vi "Compute DistanceToTarget (Modified).vi"(8 "Y Image Resolution":i32=120, 9 "X Image Resolution":i32=160, 10 "Vertical Strip":T1, 11 "Camera Type":enum16{"206", "1011", "1013"}(ring)=enum."1011") -> (0 "Distance to Wall (ft)":dbl, 2 "Target Center (-1 to 1)":cluster{"X":dbl, "Y":dbl}, 3 "Distance to Goal Wall (ft)":dbl)   [LabVIEW 2013]
doc: "Using the camera lens information and the real world size of the target, use trig and ratios to determine the distance to the target. Also returns the location relative to the image center in a (-1 , 1) coordinate system that may be useful for steering the robot."
panel:
  in  "Slope correction (goal wall)":dbl=0.365
  in  "Offset (goal wall)":dbl=0.889
  in  "Slope correction":dbl=0.87
  in  "Offset":dbl=0.835
  in  "Camera view angles":dbl[](array[numeric])=[41.7, 37.4, 49.0]
  # "37.4 default for M1011"
  # "Axis 206\nAxis M1011\nAxis M1013"
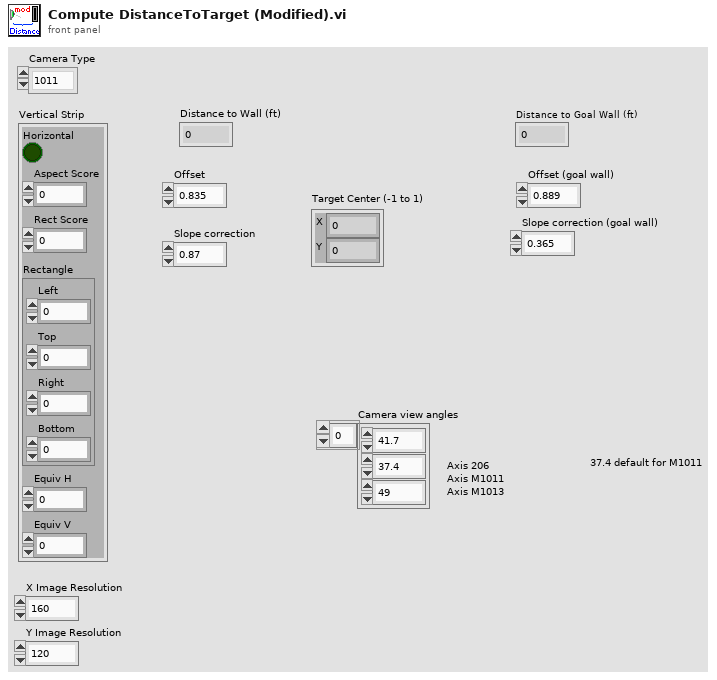
[diagram p1: front panel]
types:
  T1 = cluster{"Horizontal":bool, "Aspect Score":dbl, "Rect Score":dbl, "Rectangle":cluster{"Left":dbl, "Top":dbl, "Right":dbl, "Bottom":dbl}, "Equiv H":dbl, "Equiv V":dbl}
  T2 = cluster{"X Image Resolution":i32, "Y Image Resolution":i32}
  T3 = cluster{"X Image Resolution":dbl, "Y Image Resolution":dbl}
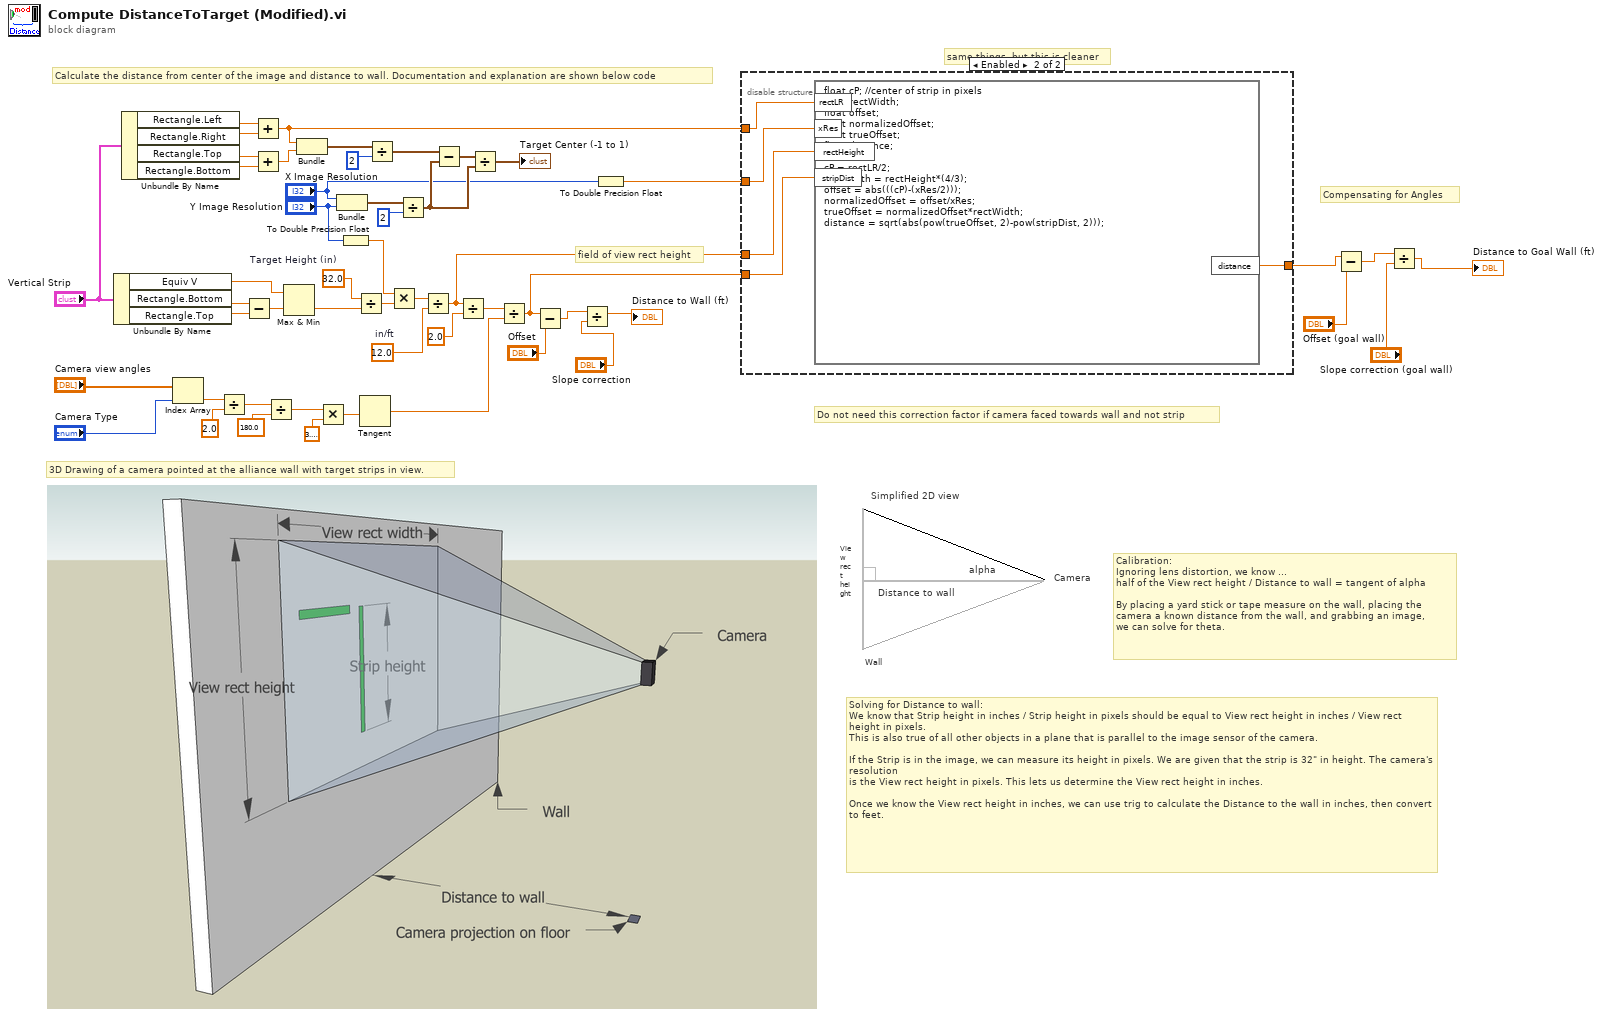
[diagram p0: block diagram]
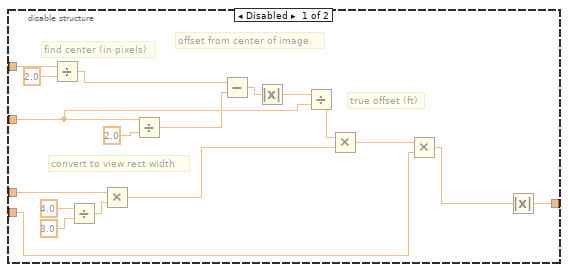
[diagram p2: hidden frame]
diagram:
  w21 = 12.0  # in/ft
  w25 = 32.0  # Target Height (in)
  # "Do not need this correction factor if camera faced towards wall and not strip"
  # "Compensating for Angles"
  # "same things, but this is cleaner"
  # "field of view rect height"
  # "Wall"
  # "Camera"
  # "Simplified 2D view"
  # "Solving for Distance to wall:\nWe know that Strip height in inches / Strip height in pixels should be equal to View rect height in inches / View rect height in pixels.\nThis is also true of all other objects in a plane that is parallel to the image sensor of the camera.\n\nIf the Strip is in the image, we can measure its height in pixels. We are given that the strip is 32\" in height. The camera's resolution\nis the View rect height in pixels. This lets us determine the View rect height in inches.\n\nOnce we know the View rect height in inches, we can use trig to calculate the Distance to the wall in inches, then convert to feet."
  # "3D Drawing of a camera pointed at the alliance wall with target strips in view."
  # "Distance to wall"
  # "View rect height"
  # "alpha"
  # "Calibration:\nIgnoring lens distortion, we know ...\nhalf of the View rect height / Distance to wall = tangent of alpha\n\nBy placing a yard stick or tape measure on the wall, placing the\ncamera a known distance from the wall, and grabbing an image,\nwe can solve for theta."
  # "Calculate the distance from center of the image and distance to wall. Documentation and explanation are shown below code"
  n1 = Unbundle By Name("Vertical Strip") -> ("Equiv V"=w27:dbl, "Rectangle.Bottom"=w42:dbl, "Rectangle.Top"=w41:dbl)
  n2 = Unbundle By Name("Vertical Strip") -> ("Rectangle.Left"=w36:dbl, "Rectangle.Right"=w37:dbl, "Rectangle.Top"=w39:dbl, "Rectangle.Bottom"=w38:dbl)
  n3 = Index Array(array="Camera view angles", index="Camera Type") -> (element=w48:dbl)
  n4 = Divide(x=w48, y=2.0) -> (x/y=w45:dbl)
  n5 = Subtract(x=w42, y=w41) -> (x-y=w26:dbl)
  n6 = Add(x=w36, y=w37) -> (x+y=w14:dbl)
  n7 = Add(x=w39, y=w38) -> (x+y=w34:dbl)
  n8 = Divide(x=w45, y=180.0) -> (x/y=w44:dbl)
  n9 = Max & Min(x=w27, y=w26) -> (min(x,y)=w10:dbl)  [unwired: 1 out]
  n10 = Bundle(w14, w34) -> (w31:cluster{dbl, dbl})  [unwired: 1 in]
  n11 = Multiply(x=w44, y=3.141592653589793) -> (x*y=w46:dbl)
  n12 = Bundle("X Image Resolution"="X Image Resolution", "Y Image Resolution"="Y Image Resolution") -> (w33:T2)  [unwired: 1 in]
  n13 = To Double Precision Float(number="Y Image Resolution") -> (double precision float=w11:dbl)
  n14 = Divide(x=w25, y=w10) -> (x/y=w24:dbl)
  n15 = Tangent(1:w46) -> (0:w18:dbl)
  n16 = Divide(x=w31, y=2) -> (x/y=w17:cluster{dbl, dbl})
  n17 = Multiply(x=w11, y=w24) -> (x*y=w22:dbl)
  n18 = Divide(x=w33, y=2) -> (x/y=w29:T3)
  n19 = Divide(x=w22, y=w21) -> (x/y=w15:dbl)
  n20 = Subtract(x=w17, y=w29) -> (x-y=w30:cluster{dbl, dbl})
  n21 = Divide(x=w15, y=2.0) -> (x/y=w19:dbl)
  n22 = Divide(x=w30, y=w29) -> (x/y=→"Target Center (-1 to 1)":cluster{dbl, dbl})
  n23 = Divide(x=w19, y=w18) -> (x/y=w12:dbl)
  n24 = Subtract(x=w12, y="Offset") -> (x-y=w7:dbl)
  n25 = Divide(x=w7, y="Slope correction") -> (x/y=→"Distance to Wall (ft)":dbl)
  n26 = To Double Precision Float(number="X Image Resolution") -> (double precision float=w13:dbl)
  n27 = disable-structure shown="Enabled" {
    disable-tunnel: [w52 w71] -> w5
    disable-tunnel: w15 -> [w57 w73]
    disable-tunnel: w14 -> [w56 w74]
    disable-tunnel: w13 -> [w55 w72]
    disable-tunnel: w12 -> [w53 w70]
    frame Disabled {
      # "true offset (ft)"
      # "offset from center of image"
      # "find center (in pixels)"
      # "convert to view rect width"
      n28 = Divide(x=w56, y=2.0) -> (x/y=w58:dbl)
      n29 = Divide(x=4.0, y=3.0) -> (x/y=w69:dbl)
      n30 = Multiply(x=w57, y=w69) -> (x*y=w65:dbl)
      n31 = Divide(x=w55, y=2.0) -> (x/y=w63:dbl)
      n32 = Subtract(x=w58, y=w63) -> (x-y=w62:dbl)
      n33 = Absolute Value(x=w62) -> (abs(x)=w61:dbl)
      n34 = Divide(x=w61, y=w55) -> (x/y=w59:dbl)
      n35 = Multiply(x=w59, y=w65) -> (x*y=w60:dbl)
      n36 = Multiply(x=w60, y=w53) -> (x*y=w54:dbl)
      n37 = Absolute Value(x=w54) -> (abs(x)=w52:dbl)
    }
    frame Enabled {
      n38 = formula code="float cP; //center of strip in pixels\nfloat rectWidth;\nfloat offset;\nfloat normalizedOffset;\nfloat trueOffset;\nfloat distance;\n\ncP = rectLR/2;\nrectWidth = rectHeight*(4/3);\noffset = abs(((cP)-(xRes/2)));\nnormalizedOffset = offset/xRes;\ntrueOffset = normalizedOffset*rectWidth;\ndistance = sqrt(abs(pow(trueOffset, 2)-pow(stripDist, 2)));"("rectLR"=w74, "rectHeight"=w73, "xRes"=w72, "stripDist"=w70) -> ("distance"=w71:dbl)
    }
  }
  n39 = Subtract(x=w5, y="Offset (goal wall)") -> (x-y=w2:dbl)
  n40 = Divide(x=w2, y="Slope correction (goal wall)") -> (x/y=→"Distance to Goal Wall (ft)":dbl)
